vi "RT Package Installer.vi"() -> ()   [LabVIEW 2018]
uses:
  <vilib>/nisyscfg/Software 1.2.ctl
  <vilib>/nisyscfg/Component Type.ctl
  <vilib>/WebDAVClient/Advanced/Put File.vi
  <vilib>/nisyscfg/Get Installed Components.vi
  <vilib>/nisyscfg/nisyscfg.lvlib
  <vilib>/WebDAVClient/NI_WebDAV.lvlib
  <resource>/objmgr/nisysapi.rc
panel:
  in  "Tab Control":enum32{"From Feed", "Local File"}(tab)
  in  "Package Name":string
  in  "Path":path
  out "Installed Packages":string[][](table)
  in  "Password":string
  in  "Target (localhost)":refnum<k21>="localhost"
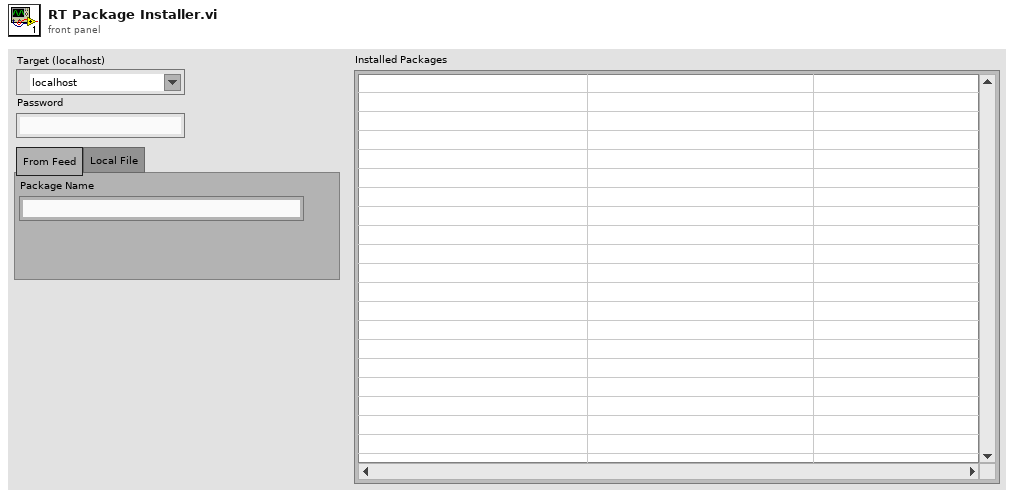
[diagram p1: front panel]
types:
  T1 = typedef "nisyscfg.lvlib/Software 1.2.ctl" = cluster{"title":string, "description":string, "ID":string, "version":string, "component type":T2}
  T2 = typedef "nisyscfg.lvlib/Component Type.ctl" = u32
  T3 = typedef "NI_WebDAV.lvlib/SessionHandle.ctl" = refnum<k1>
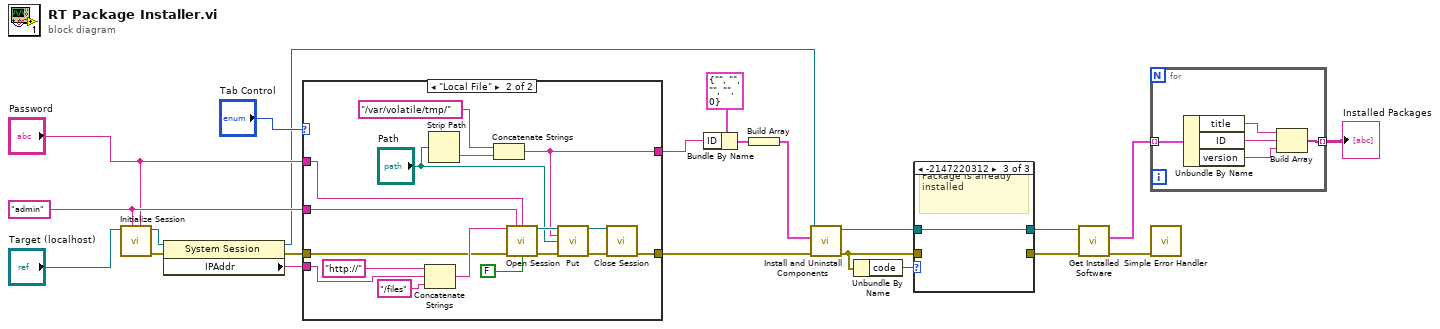
[diagram p0: block diagram]
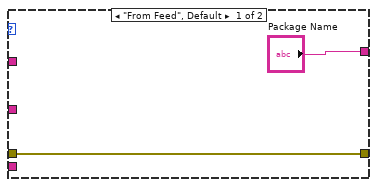
[diagram p4: hidden frame]
diagram:
  w14 = "admin" ("User Name")
  n1 = call <vilib>:"Initialize Session.vi"("Password"="Password", "User Name"=w14, "Target (localhost)"="Target (localhost)") -> ("error out"=w11:errorcluster, "Session out"=w12:refnum<k21>)  [unwired: 7 in]
  n2 = property class="System Session"(reference=w12, error in=w11) -> (reference out=w7:refnum<k21>, error out=w9:errorcluster, "IPAddr"=w10:string)
  n3 = case shown="\"Local File\"" "Tab Control" {
    tunnel: ["Package Name" w28] -> w16
    tunnel: w10 -> [_ w40]
    tunnel: w14 -> [_ w37]
    tunnel: "Password" -> [_ w36]
    tunnel: w9 -> [w23 w27]
    tunnel: [w23 w26] -> w8
    frame "From Feed", Default {
    }
    frame "Local File" {
      n4 = Concatenate Strings("http://" ("string"), w40, "/files" ("string")) -> (w38:string)
      n5 = Strip Path(path="Path") -> (name=w29:string)  [unwired: 1 out]
      n6 = Concatenate Strings("/var/volatile/tmp/" ("relative uri"), w29) -> (w28:string)
      n7 = call <vilib>:"Open Session.vi"("host uri prefix"=w38, "username"=w37, "password"=w36, "error in (no error)"=w27, "verify server?"=FALSE) -> ("session handle out"=w35:T3, "error out"=w33:errorcluster)  [unwired: 9 in]
      n8 = call-poly <vilib>:"Put.vi"("session handle"=w35, "relative uri"=w28, "local file path"="Path", "error in (no error)"=w33) -> ("session handle out"=w34:T3, "error out"=w32:errorcluster)  [unwired: 9 in, 1 out]
      n9 = call <vilib>:"Close Session.vi"("session handle"=w34, "error in (no error)"=w32) -> ("error out"=w26:errorcluster)  [unwired: 13 in]
    }
  }
  n10 = Bundle By Name(cluster=T1 {"title"="", "description"="", "ID"="", "version"="", "component type"=0} ("Software"), "ID"=w16) -> (w21:T1)
  n11 = Build Array(w21) -> (w20:T1[])
  n12 = call <vilib>:"Install and Uninstall Components.vi"("error in (no error)"=w8, "Software Components to Install"=w20, "Session in"=w7) -> ("error out"=w2:errorcluster, "Session out"=w5:refnum<k21>)  [unwired: 6 in, 1 out]
  n13 = Unbundle By Name(w2) -> ("code"=w3:i32)
  n14 = case shown="-2147220312" w3 {
    tunnel: [w42 w44 _] -> w6
    tunnel: w5 -> [w43 w45 w46]
    tunnel: [w43 w45 w46] -> w4
    tunnel: w2 -> [w42 w44 _]
    frame 0 {
    }
    frame 1, Default {
    }
    frame -2147220312 {
      # "Package is already installed"
    }
  }
  n15 = call-poly <vilib>:"Get Installed Software.vi"("error in (no error)"=w6, "Session in"=w4) -> ("error out"=w1:errorcluster, "Software Components"=w19:T1[])  [unwired: 7 in, 1 out]
  n16 = for {
    tunnel: w19 -> [w51] mode=indexing
    tunnel: [w48] -> w18 mode=indexing
    n17 = Unbundle By Name(w51) -> ("title"=w50:string, "ID"=w49:string, "version"=w47:string)
    n18 = Build Array(w50, w49, w47) -> (w48:string[])
  }
  "Installed Packages" <- w18
  n19 = call <vilib>:"Simple Error Handler.vi"("error in (no error)"=w1) -> ()  [unwired: 4 in, 5 out]
